vi "SPI_Set_GPIOs.vi"(1 "High IOs Config":T2, 2 "CSDisableStates":T1, 3 "Handle":u32) -> (0 "FTC_Status":u32)   [LabVIEW 2010]
uses:
  FTCSPI.dll
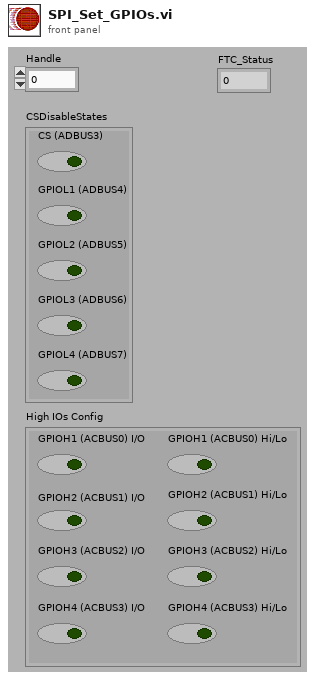
[diagram p1: front panel]
types:
  T1 = cluster{"CS (ADBUS3)":bool, "GPIOL1 (ADBUS4)":bool, "GPIOL2 (ADBUS5)":bool, "GPIOL3 (ADBUS6)":bool, "GPIOL4 (ADBUS7)":bool}
  T2 = cluster{"GPIOH1 (ACBUS0) I/O":bool, "GPIOH1 (ACBUS0) Hi/Lo":bool, "GPIOH2 (ACBUS1) I/O":bool, "GPIOH2 (ACBUS1) Hi/Lo":bool, "GPIOH3 (ACBUS2) I/O":bool, "GPIOH3 (ACBUS2) Hi/Lo":bool, "GPIOH4 (ACBUS3) I/O":bool, "GPIOH4 (ACBUS3) Hi/Lo":bool}
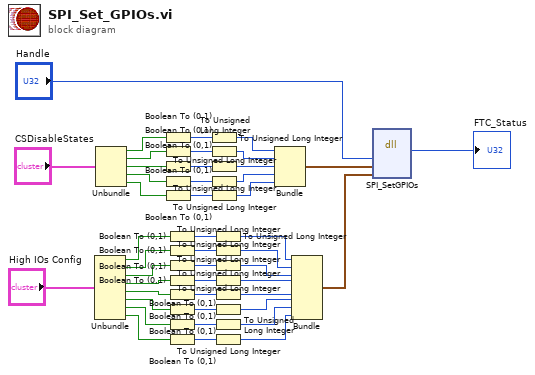
[diagram p0: block diagram]
diagram:
  n1 = Unbundle("High IOs Config") -> ("GPIOH1 (ACBUS0) I/O"=w34:bool, "GPIOH1 (ACBUS0) Hi/Lo"=w33:bool, "GPIOH2 (ACBUS1) I/O"=w32:bool, "GPIOH2 (ACBUS1) Hi/Lo"=w31:bool, "GPIOH3 (ACBUS2) I/O"=w30:bool, "GPIOH3 (ACBUS2) Hi/Lo"=w29:bool, "GPIOH4 (ACBUS3) I/O"=w28:bool, "GPIOH4 (ACBUS3) Hi/Lo"=w27:bool)
  n2 = Unbundle("CSDisableStates") -> ("CS (ADBUS3)"=w11:bool, "GPIOL1 (ADBUS4)"=w10:bool, "GPIOL2 (ADBUS5)"=w9:bool, "GPIOL3 (ADBUS6)"=w8:bool, "GPIOL4 (ADBUS7)"=w7:bool)
  n3 = Boolean To (0,1)(Boolean=w11) -> (0, 1=w16:i16)
  n4 = Boolean To (0,1)(Boolean=w10) -> (0, 1=w15:i16)
  n5 = Boolean To (0,1)(Boolean=w9) -> (0, 1=w14:i16)
  n6 = Boolean To (0,1)(Boolean=w8) -> (0, 1=w13:i16)
  n7 = Boolean To (0,1)(Boolean=w7) -> (0, 1=w12:i16)
  n8 = Boolean To (0,1)(Boolean=w34) -> (0, 1=w42:i16)
  n9 = Boolean To (0,1)(Boolean=w33) -> (0, 1=w41:i16)
  n10 = Boolean To (0,1)(Boolean=w32) -> (0, 1=w40:i16)
  n11 = Boolean To (0,1)(Boolean=w31) -> (0, 1=w39:i16)
  n12 = Boolean To (0,1)(Boolean=w30) -> (0, 1=w38:i16)
  n13 = Boolean To (0,1)(Boolean=w29) -> (0, 1=w37:i16)
  n14 = Boolean To (0,1)(Boolean=w28) -> (0, 1=w36:i16)
  n15 = Boolean To (0,1)(Boolean=w27) -> (0, 1=w35:i16)
  n16 = To Unsigned Long Integer(number=w16) -> (unsigned 32bit integer=w6:u32)
  n17 = To Unsigned Long Integer(number=w15) -> (unsigned 32bit integer=w5:u32)
  n18 = To Unsigned Long Integer(number=w14) -> (unsigned 32bit integer=w4:u32)
  n19 = To Unsigned Long Integer(number=w13) -> (unsigned 32bit integer=w3:u32)
  n20 = To Unsigned Long Integer(number=w12) -> (unsigned 32bit integer=w2:u32)
  n21 = To Unsigned Long Integer(number=w42) -> (unsigned 32bit integer=w26:u32)
  n22 = To Unsigned Long Integer(number=w41) -> (unsigned 32bit integer=w25:u32)
  n23 = To Unsigned Long Integer(number=w40) -> (unsigned 32bit integer=w24:u32)
  n24 = To Unsigned Long Integer(number=w39) -> (unsigned 32bit integer=w23:u32)
  n25 = To Unsigned Long Integer(number=w38) -> (unsigned 32bit integer=w22:u32)
  n26 = To Unsigned Long Integer(number=w37) -> (unsigned 32bit integer=w21:u32)
  n27 = To Unsigned Long Integer(number=w36) -> (unsigned 32bit integer=w20:u32)
  n28 = To Unsigned Long Integer(number=w35) -> (unsigned 32bit integer=w19:u32)
  n29 = Bundle(w6, w5, w4, w3, w2) -> (w1:cluster{u32, u32, u32, u32, u32})  [unwired: 1 in]
  n30 = Bundle(w26, w25, w24, w23, w22, w21, w20, w19) -> (w18:cluster{u32, u32, u32, u32, u32, u32, u32, u32})  [unwired: 1 in]
  n31 = dll-call lib="C:/Users/Administrator/Documents/GitHub/labview/FPGA/FTCSPI.dll" fn="SPI_SetGPIOs"("Handle"="Handle", w1, w18) -> ("FTC_Status"=→"FTC_Status":u32)  [unwired: 6 in, 2 out]
